vi "Analysis prog.vi"() -> ()   [LabVIEW 2012]
panel:
  out "Histogram 3":dynamicdata(graph) caption="Histogram"
  out "Histogram 2":dynamicdata(graph) caption="Histogram"
  out "Numeric":i32
  in  "stop":bool
  out "Histogram":dynamicdata(graph)
  out "Waveform Graph":waveform(dbl)(graph)
  out "Array":dbl[](array[numeric]) format="%.2f"
  # "Analysis program to crosscheck the root analysis (very slow)"
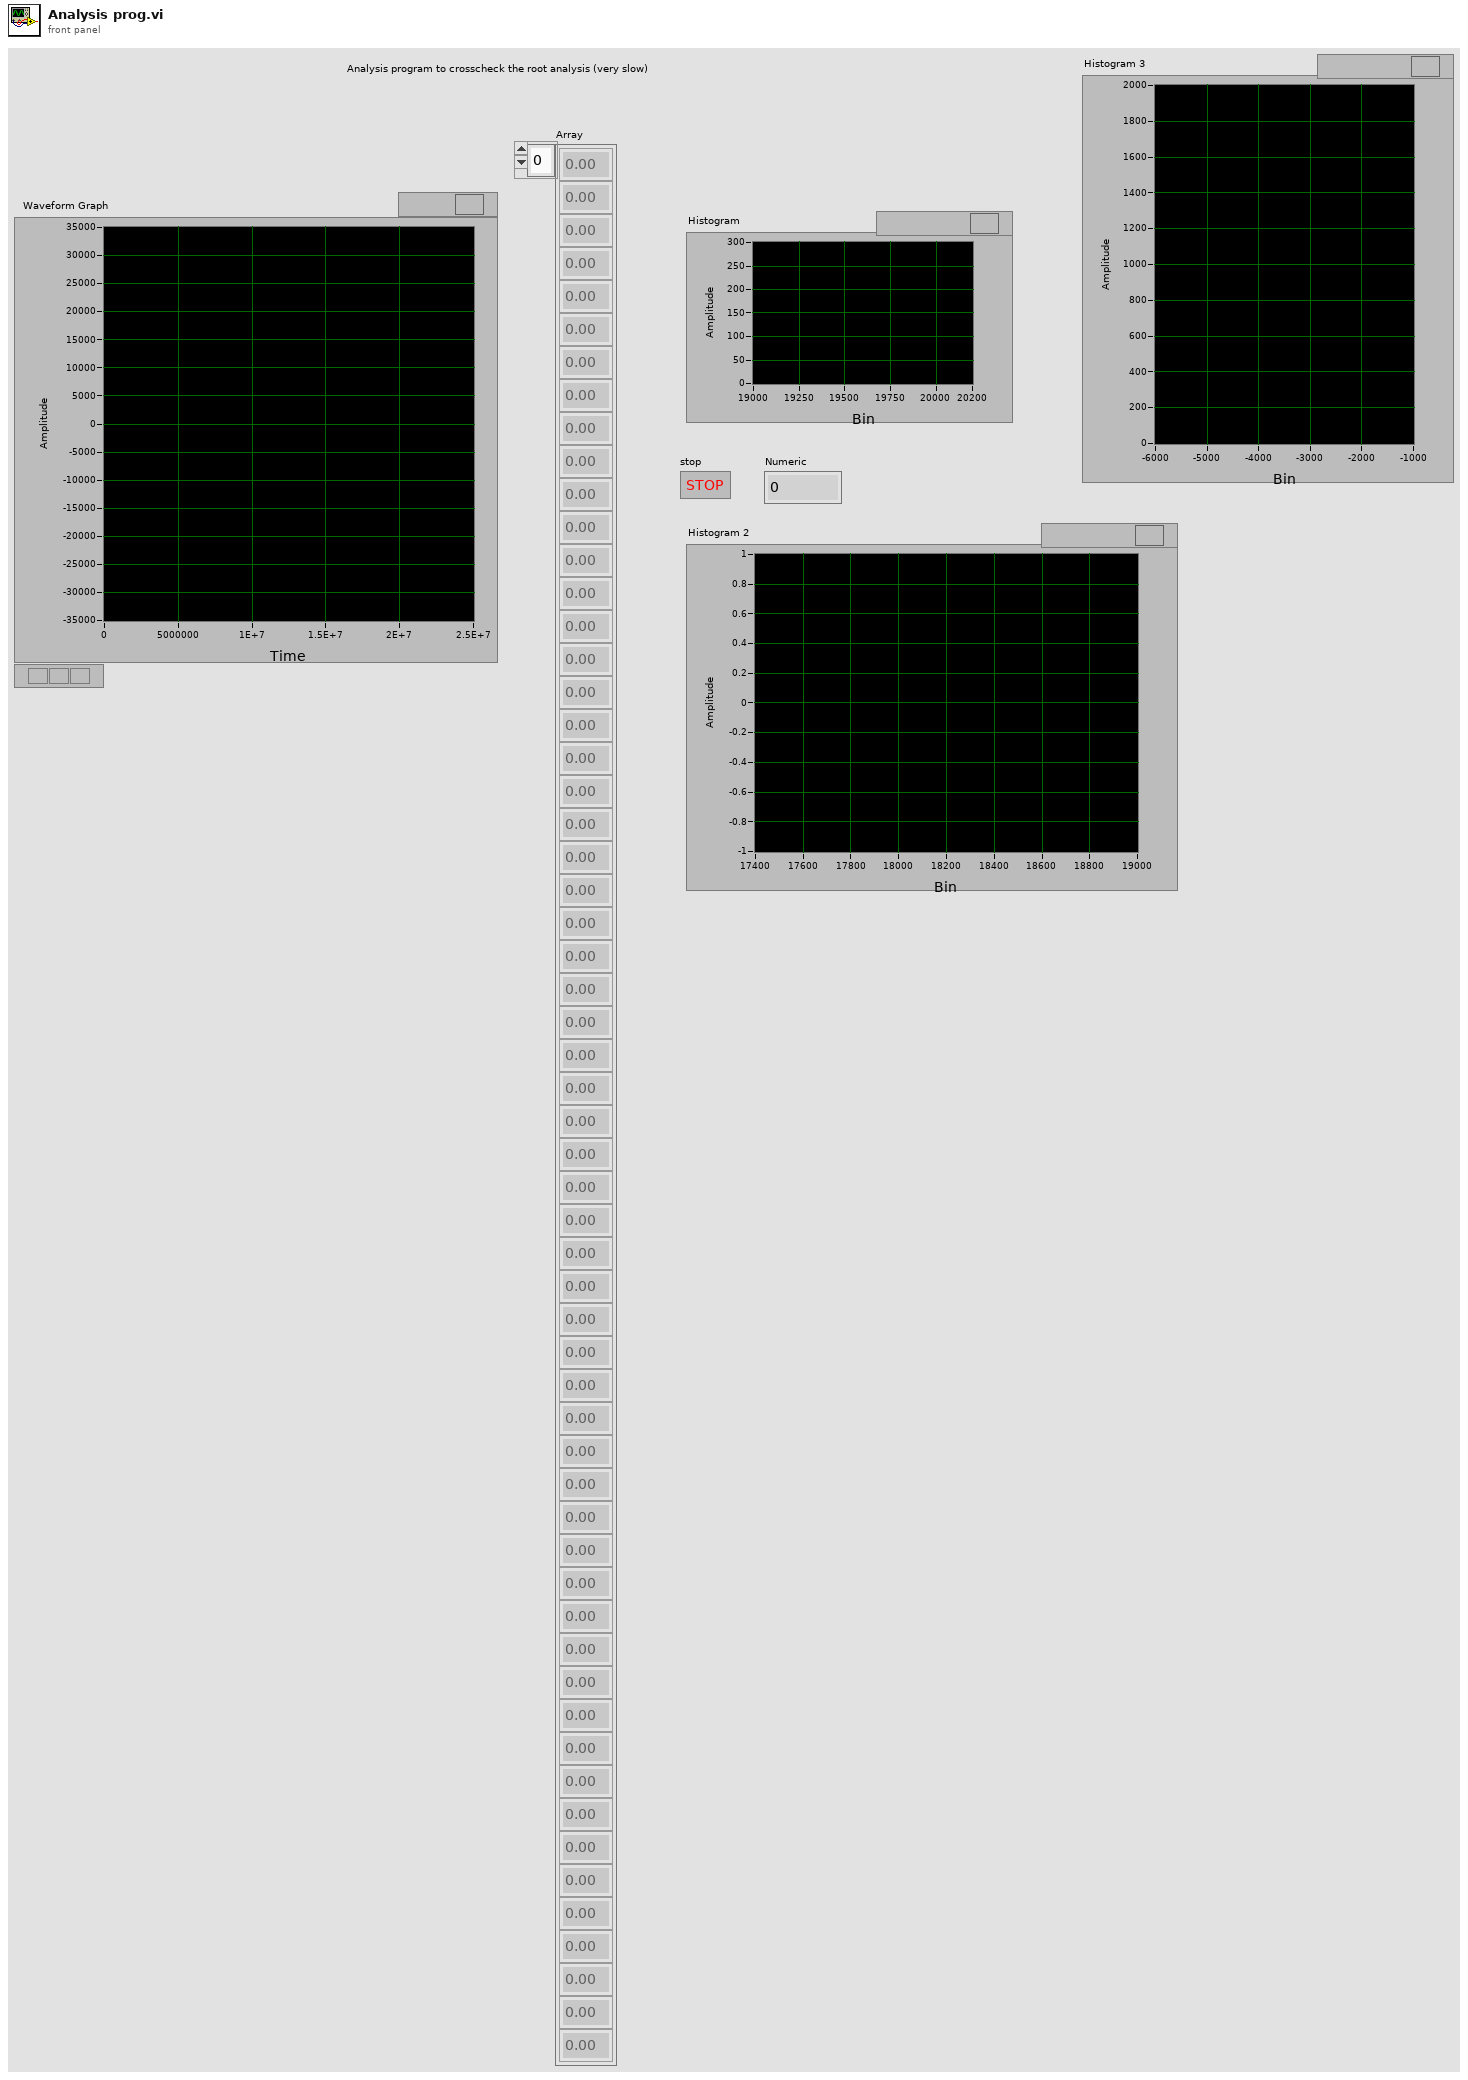
[diagram p1: front panel]
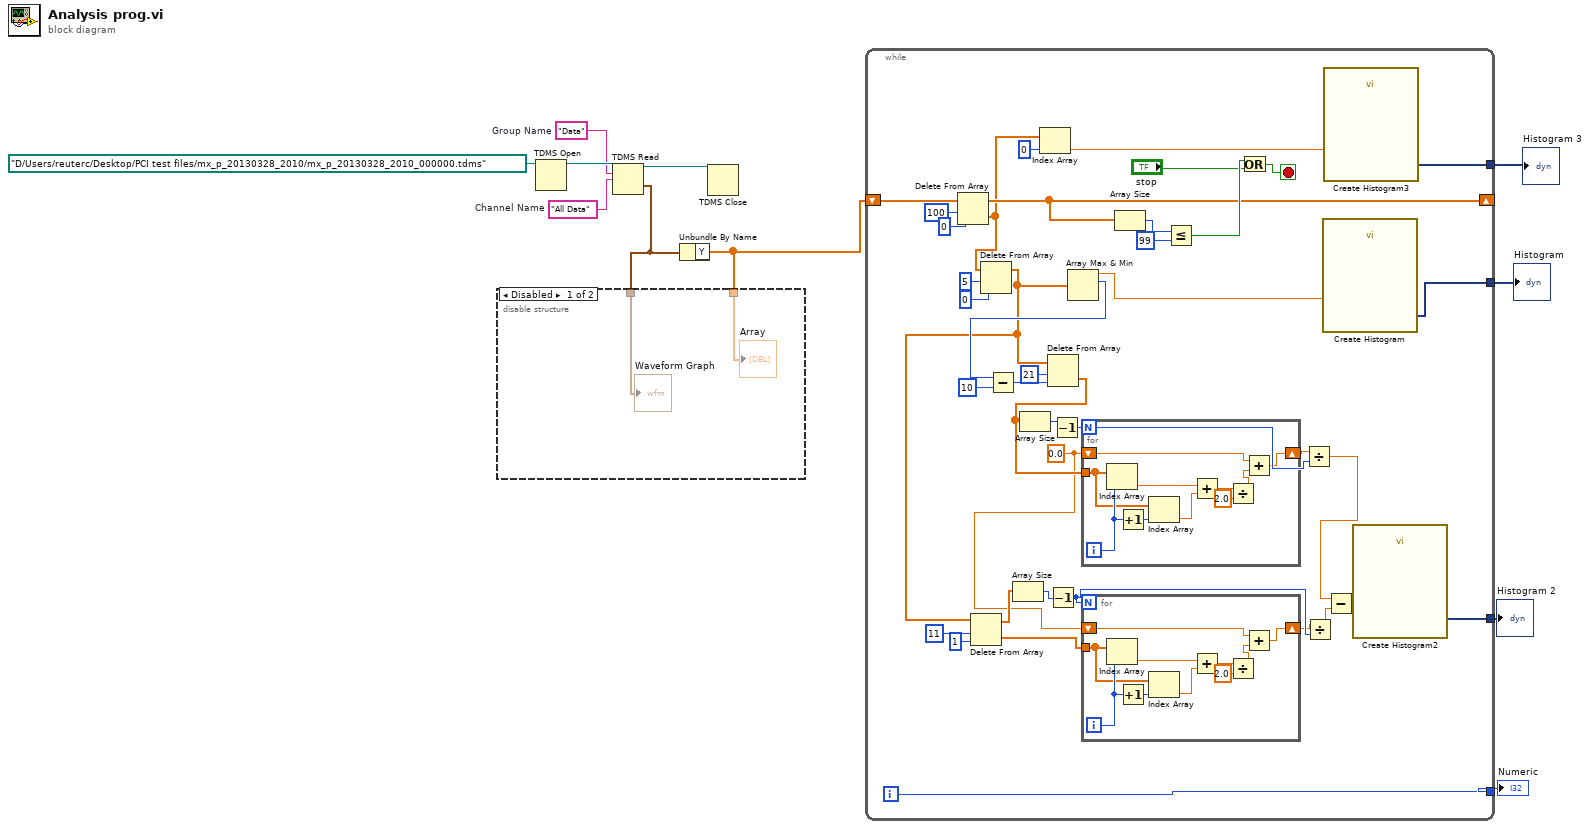
[diagram p0: block diagram]
diagram:
  w7 = "Data"  # Group Name
  w8 = "All Data"  # Channel Name
  n1 = TDMS Open(11:path "D:/Users/reuterc/Desktop/PCI test files/mx_p_20130328_2010/mx_p_20130328_2010_000000.tdms" ("file path")) -> (3:w10:refnum<k34>)  [unwired: 5 in, 1 out]
  n2 = TDMS Read(0:w10, 5:w7, 7:w8) -> (4:w9:refnum<k34>, 10:w6:waveform(dbl))  [unwired: 5 in, 4 out]
  n3 = Unbundle By Name(w6) -> ("Y"=w1:dbl[])
  n4 = disable-structure shown="Disabled" {
    disable-tunnel: w6 -> [w13 _]
    disable-tunnel: w1 -> [w12 _]
    frame Disabled {
      "Array" <- w12
      "Waveform Graph" <- w13
    }
    frame Enabled {
    }
  }
  n5 = TDMS Close(11:w9) -> ()  [unwired: 1 in, 2 out]
  n6 = while {
    shift-right: [w19] -> _
    shift-left: w1 -> [w52]
    tunnel: [w47] -> w5
    tunnel: [w34] -> w4
    tunnel: [w33] -> w3
    tunnel: [w15] -> w2
    i -> [w34]
    stop <- w44 stop-if-true
    w21 = 0.0
    n7 = Delete From Array(array=w52, length=100, index=0) -> (deleted portion=w18:dbl[], array with subset deleted=w19:dbl[])
    n8 = Delete From Array(array=w18, length=5, index=0) -> (array with subset deleted=w32:dbl[])  [unwired: 1 out]
    n9 = Delete From Array(array=w32, length=11, index=1) -> (deleted portion=w22:dbl[], array with subset deleted=w29:dbl[])
    n10 = Array Size(array=w29) -> (size(s)=w14:i32)
    n11 = Index Array(array=w18, index=0) -> (element=w16:dbl)
    n12 = Decrement(x=w14) -> (x-1=w25:i32)
    n13 = Array Max & Min(array=w32) -> (max value=w48:dbl, max index (indices)=w39:i32)  [unwired: 2 out]
    n14 = Subtract(x=w39, y=10) -> (x-y=w40:i32)
    n15 = Delete From Array(array=w32, length=21, index=w40) -> (deleted portion=w35:dbl[])  [unwired: 1 out]
    n16 = Array Size(array=w35) -> (size(s)=w36:i32)
    n17 = Decrement(x=w36) -> (x-1=w27:i32)
    n18 = for {
      N: w27 -> [_]
      tunnel: w35 -> [w70]
      shift-right: [w63] -> w28
      shift-left: w21 -> [w65]
      i -> [w71]
      n19 = Index Array(array=w70, index=w71) -> (element=w69:dbl)
      n20 = Increment(x=w71) -> (x+1=w72:i32)
      n21 = Index Array(array=w70, index=w72) -> (element=w68:dbl)
      n22 = Add(x=w69, y=w68) -> (x+y=w67:dbl)
      n23 = Divide(x=w67, y=2.0) -> (x/y=w64:dbl)
      n24 = Add(x=w65, y=w64) -> (x+y=w63:dbl)
    }
    n25 = for {
      N: w25 -> [_]
      tunnel: w22 -> [w60]
      shift-right: [w53] -> w24
      shift-left: w21 -> [w55]
      i -> [w61]
      n26 = Index Array(array=w60, index=w61) -> (element=w59:dbl)
      n27 = Increment(x=w61) -> (x+1=w62:i32)
      n28 = Index Array(array=w60, index=w62) -> (element=w58:dbl)
      n29 = Add(x=w59, y=w58) -> (x+y=w57:dbl)
      n30 = Divide(x=w57, y=2.0) -> (x/y=w54:dbl)
      n31 = Add(x=w55, y=w54) -> (x+y=w53:dbl)
    }
    n32 = Array Size(array=w19) -> (size(s)=w50:i32)
    n33 = Less Or Equal?(x=w50, y=99) -> (x <= y?=w46:bool)
    n34 = Or(x=w46, y="stop") -> (x .or. y?=w44:bool)
    n35 = Divide(x=w28, y=w27) -> (x/y=w26:dbl)
    n36 = Divide(x=w24, y=w25) -> (x/y=w20:dbl)
    n37 = call "Create Histogram"("Signal"=w48) -> ("Histogram"=w47:dynamicdata)  [unwired: 9 in, 1 out]
    n38 = call "Create Histogram3"("Signal"=w16) -> ("Histogram"=w15:dynamicdata)  [unwired: 9 in, 1 out]
    n39 = Subtract(x=w26, y=w20) -> (x-y=w23:dbl)
    n40 = call "Create Histogram2"("Signal"=w23) -> ("Histogram"=w33:dynamicdata)  [unwired: 9 in, 1 out]
  }
  "Histogram" <- w5
  "Numeric" <- w4
  "Histogram 2" <- w3
  "Histogram 3" <- w2
